vi "iBeam Laser Send Command.vi"(0 "VISA Ref":refnum<visa-resource-name>, 2 "Wait for Reply?":bool=TRUE, 7 "Command":string, 11 "Error In":errorcluster) -> (4 "VISA Ref Out":refnum<visa-resource-name>, 8 "Response":string, 15 "Error Out":errorcluster)   [LabVIEW 2020]
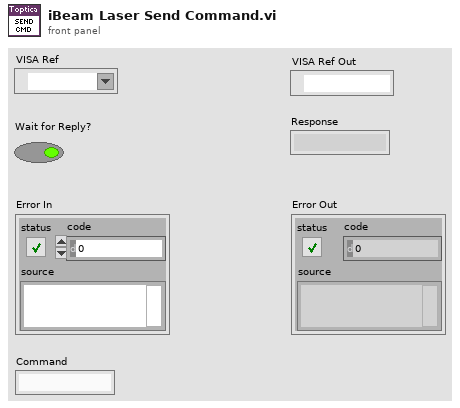
[diagram p1: front panel]
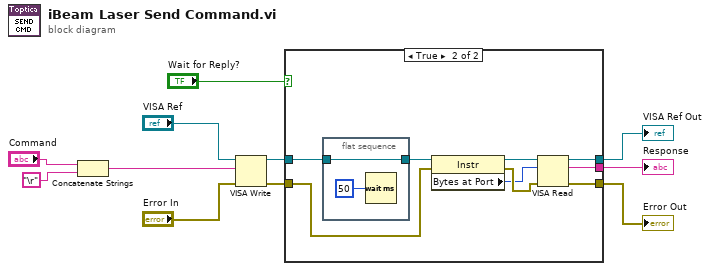
[diagram p0: block diagram]
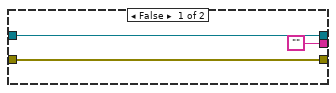
[diagram p2: hidden frame]
diagram:
  n1 = Concatenate Strings("Command", "\r") -> (w1:string)
  n2 = VISA Write(VISA resource name="VISA Ref", write buffer=w1, error in (no error)="Error In") -> (VISA resource name out=w11:refnum<visa-resource-name>, error out=w10:errorcluster)  [unwired: 1 out]
  n3 = case shown="True" "Wait for Reply?" {
    tunnel: w11 -> [w14 w19]
    tunnel: w10 -> [w13 w18]
    tunnel: [w14 w17] -> w8
    tunnel: [w13 w16] -> w7
    tunnel: ["" w15] -> w5
    frame False {
    }
    frame True {
      n4 = flat-sequence {
        tunnel: [w24] -> w22
        tunnel: w19 -> [w24]
        frame #0 {
          n5 = Wait (ms)(milliseconds to wait=u32 50) -> ()  [unwired: 1 out]
        }
      }
      n6 = property class="Instr"(reference=w22, error in=w18) -> (reference out=w20:refnum<visa-resource-name>, error out=w23:errorcluster, "Bytes at Port"=w21:u32)
      n7 = VISA Read(VISA resource name=w20, byte count=w21, error in (no error)=w23) -> (VISA resource name out=w17:refnum<visa-resource-name>, read buffer=w15:string, error out=w16:errorcluster)  [unwired: 1 out]
    }
  }
  "Response" <- w5
  "VISA Ref Out" <- w8
  "Error Out" <- w7
